vi "String Functions 1.vi"() -> ()   [LabVIEW 2015]
panel:
  in  "SubString Offset":i32
  in  "SubString Length":i32
  out "String Subset":string
  out "Welcome Message":string
  out "User Name Length":i32
  in  "User Name":string
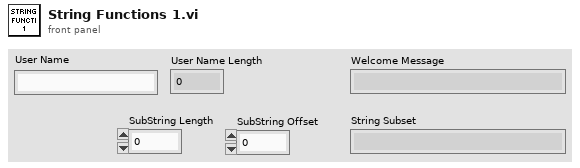
[diagram p1: front panel]
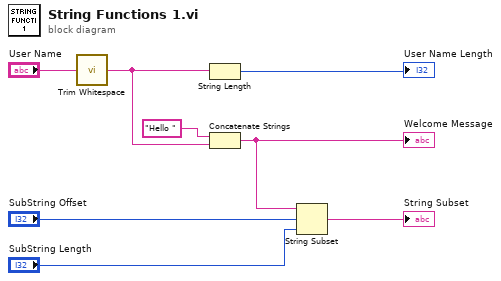
[diagram p0: block diagram]
diagram:
  n1 = call <vilib>:"Trim Whitespace.vi"("string"="User Name") -> ("trimmed string"=w5:string)  [unwired: 1 in]
  n2 = String Length(string=w5) -> (length=→"User Name Length":i32)
  n3 = Concatenate Strings "Concatenate Strings"("Hello " ("string"), w5) -> (w4:string)
  "Welcome Message" <- w4
  n4 = String Subset(string=w4, offset (0)="SubString Offset", length (rest)="SubString Length") -> (substring=→"String Subset":string)
